vi "_FPGA_HighestValueAbsI16.vi"(9 "Enable":bool, 10 "Init":bool, 11 "Value in":i16) -> (3 "Highest Value":i16)   [LabVIEW 2018]
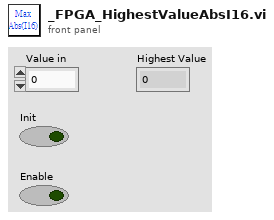
[diagram p1: front panel]
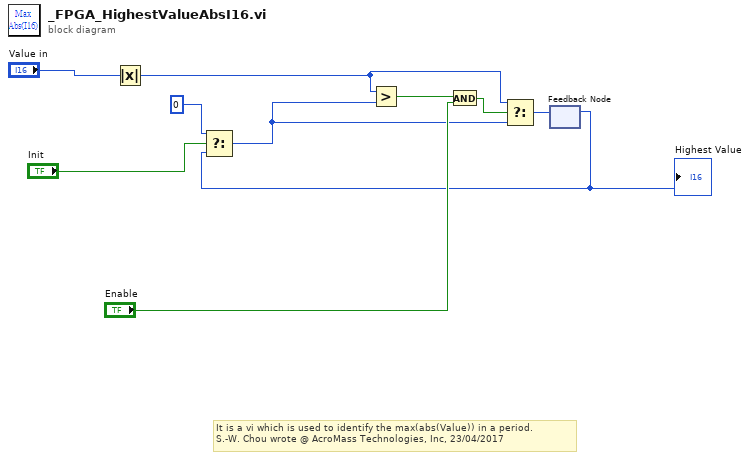
[diagram p0: block diagram]
diagram:
  # "It is a vi which is used to identify the max(abs(Value)) in a period.\nS.-W. Chou wrote @ AcroMass Technologies, Inc, 23/04/2017"
  n1 = Absolute Value(x="Value in") -> (abs(x)=w2:i16)
  n2 = feedback #1() -> (w6:i16)  [unwired: 1 in]
  "Highest Value" <- w6
  n3 = Select(t=i16 0, s="Init", f=w6) -> (s? t:f=w4:i16)
  n4 = Greater?(x=w2, y=w4) -> (0:w1:bool)
  n5 = And(x=w1, y="Enable") -> (x .and. y?=w7:bool)
  n6 = Select(t=w2, s=w7, f=w4) -> (s? t:f=w3:i16)
  n7 = feedback-in #1(w3) -> ()
